vi "SRingThreadIsOFF.vi"() -> (0 "ThreadIsOFF":u8)   [LabVIEW 2015]
uses:
  TRANCON/DLL/lwlscdll.dll
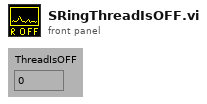
[diagram p1: front panel]
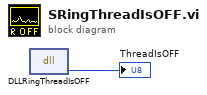
[diagram p0: block diagram]
diagram:
  n1 = dll-call lib="G:/SD/TRANCON/DLL/lwlscdll.dll" fn="DLLRingThreadIsOFF"() -> (→"ThreadIsOFF":u8)  [unwired: 3 in, 2 out]
